vi "CloseCamera.vi"(8 "error in (no error)":errorcluster, 11 "ZWO_ASI in":refnum<class "ZWO_ASI.lvclass">) -> (0 "error out":errorcluster, 3 "ZWO_ASI out":refnum<class "ZWO_ASI.lvclass">)   [LabVIEW 2023, in "ZWO_ASI.lvlib" / "ZWO_ASI.lvclass"]
uses:
  ZWO_ASI.lvclass
  ZWO_ASI.lvclass/ZWO_ASI.ctl
  <userlib>/ASICamera2_no_err/ASICamera2_no_err.lvlib
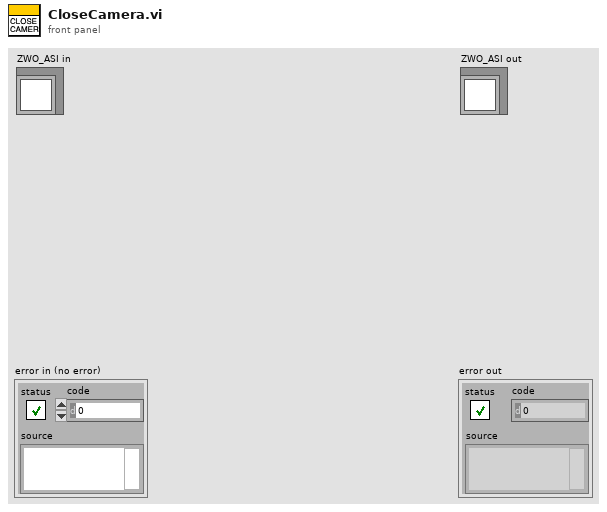
[diagram p1: front panel]
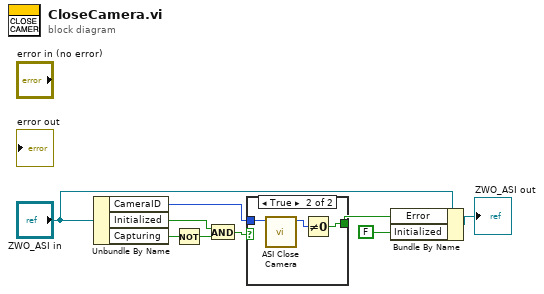
[diagram p0: block diagram]
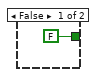
[diagram p2: hidden frame]
diagram:
  n1 = Unbundle By Name("ZWO_ASI in") -> ("CameraID"=w9:i32, "Initialized"=w7:bool, "Capturing"=w8:bool)
  n2 = Not(x=w8) -> (.not. x?=w6:bool)
  n3 = And(x=w7, y=w6) -> (x .and. y?=w5:bool)
  n4 = case shown="True" w5 {
    tunnel: w9 -> [_ w13]
    tunnel: [FALSE w11] -> w3
    frame False {
    }
    frame True {
      n5 = call <userlib>:"ASI Close Camera.vi"("iCameraID"=w13) -> ("function return"=w12:i32)  [unwired: 10 in]
      n6 = Not Equal To 0?(x=w12) -> (x != 0?=w11:bool)
    }
  }
  n7 = Bundle By Name(cluster="ZWO_ASI in", "Error"=w3, "Initialized"=FALSE) -> (→"ZWO_ASI out":refnum<class "ZWO_ASI.lvclass">)
